vi "FFT (SubVI).vi"(9 "Array":cdb[](array[numeric]), 10 "Sample Rate":dbl, 11 "FM  Frequency":dbl) -> (3 "FM Spectrum":cluster{dbl[], dbl[]}[](graph))   [LabVIEW 2013]
uses:
  <vilib>/Analysis/1siggen.llb/Ramp Pattern by Samples.vi
  <vilib>/Analysis/2dsp.llb/Complex FFT.vi
  <vilib>/Analysis/NI_AALPro.lvlib
  <vilib>/Analysis/NI_AALBase.lvlib
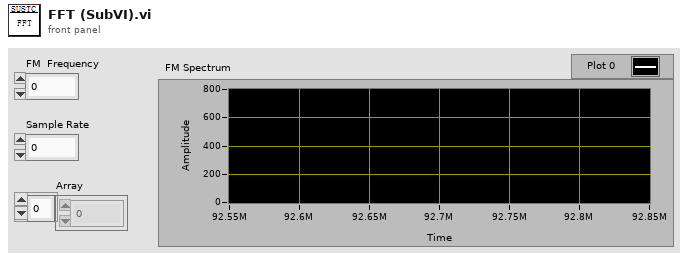
[diagram p1: front panel]
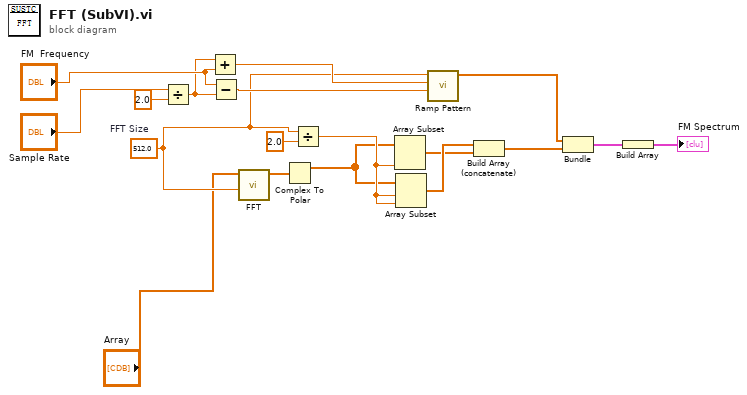
[diagram p0: block diagram]
diagram:
  w13 = 512.0  # FFT Size
  n1 = Divide(x="Sample Rate", y=2.0) -> (x/y=w14:dbl)
  n2 = Add(x=w14, y="FM  Frequency") -> (x+y=w17:dbl)
  n3 = Subtract(x="FM  Frequency", y=w14) -> (x-y=w16:dbl)
  n4 = call-poly <vilib>:"FFT.vi"("FFT size"=w13, "X"="Array") -> ("FFT {X}"=w1:cdb[])  [unwired: 8 in, 1 out]
  n5 = Complex To Polar(r * e^(i*theta)=w1) -> (r=w5:dbl[])  [unwired: 1 out]
  n6 = Divide(x=w13, y=2.0) -> (x/y=w7:dbl)
  n7 = Array Subset(array=w5, length=w7) -> (w3:dbl[])  [unwired: 1 in]
  n8 = Array Subset(array=w5, index=w7, length=w7) -> (w4:dbl[])
  n9 = call-poly <vilib>:"Ramp Pattern.vi"("start"=w16, "end"=w17, "samples"=w13) -> ("Ramp Pattern"=w12:dbl[])  [unwired: 7 in, 1 out]
  n10 = Build Array (concatenate)(w4, w3) -> (w10:dbl[])
  n11 = Bundle("Ramp Pattern"=w12, w10) -> (w8:cluster{"Ramp Pattern":dbl[], dbl[]})  [unwired: 1 in]
  n12 = Build Array(w8) -> (→"FM Spectrum":cluster{"Ramp Pattern":dbl[], dbl[]}[])
